vi "Get Item Data.vi"(8 "error in (no error)":errorcluster, 11 "Item Reference in":T2 format="%.0x") -> (0 "error out":errorcluster, 2 "Item Info":T1={"Name"="", "TagGUID"="", "TypeGUID"="", "Enable"=TRUE}, 3 "Item Reference out":T2 format="%.0x", 4 "found":bool)   [LabVIEW 2013, in "Hierarchy Framework.lvlib" / "Item.lvclass"]
doc: "Returns information about the item specified by <B>Item Reference in</B>, including the name of the item,and whether the item is Enable."
uses:
  Item.lvclass
  Ctls/Item Reference.ctl
  Ctls/Item Info.ctl
  Generic/Generic.lvclass
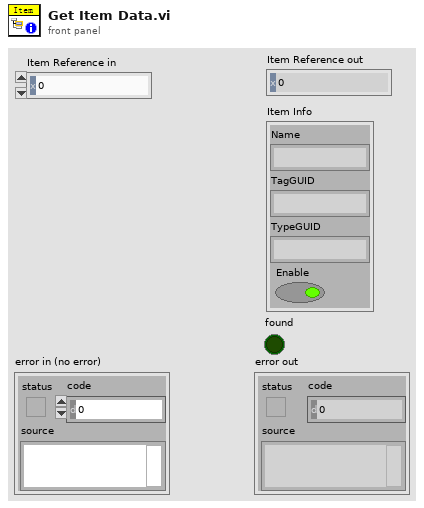
[diagram p1: front panel]
types:
  T1 = typedef "Hierarchy Framework.lvlib/Item.lvclass/Item Info.ctl" = cluster{"Name":string, "TagGUID":string, "TypeGUID":string, "Enable":bool}
  T2 = typedef "Hierarchy Framework.lvlib/Item.lvclass/Item Reference.ctl" = u64
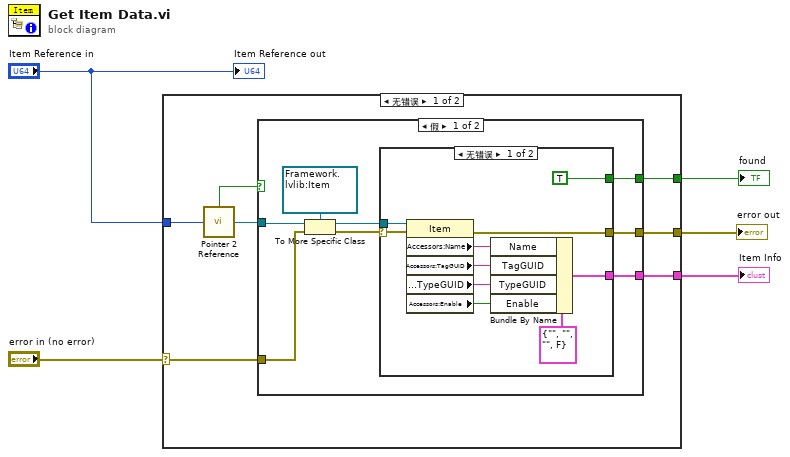
[diagram p0: block diagram]
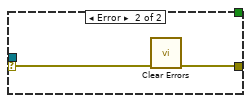
[diagram p2: hidden frame]
diagram:
  n1 = case shown="无错误" "error in (no error)" {
    selector: "error in (no error)" -> [w11 w34]
    tunnel: "Item Reference in" -> [w10 _]
    tunnel: [w12 w34] -> w4
    tunnel: [w7 _] -> w2
    tunnel: [w6 _] -> w1
    frame No Error {
      n2 = call "Pointer 2 Reference.vi"("Pointer"=w10) -> ("Not A Refnum?"=w9:bool, "Generic Reference"=w8:refnum<data-value>)
      n3 = case shown="假" w9 {
        tunnel: w11 -> [w19 w33]
        tunnel: [w16 w33] -> w12
        tunnel: w8 -> [w20 _]
        tunnel: [w15 _] -> w7
        tunnel: [w14 _] -> w6
        frame False {
          n4 = To More Specific Class(target class=refnum<data-value> refnum ("Item"), reference=w20, error in=w19) -> (specific class reference=w17:refnum<data-value>, error out=w13:errorcluster)
          n5 = case shown="无错误" w13 {
            selector: w13 -> [w21 w32]
            tunnel: w17 -> [w30 _]
            tunnel: [w29 w31] -> w16
            tunnel: [TRUE _] -> w15
            tunnel: [w23 _] -> w14
            frame No Error {
              n6 = property class="Item"(reference=w30, error in=w21) -> (error out=w29:errorcluster, "Accessors:Name"=w26:string, "Accessors:TagGUID"=w25:string, "Accessors:TypeGUID"=w22:string, "Accessors:Enable"=w24:bool)  [unwired: 1 out]
              n7 = Bundle By Name(cluster=T1 {"Name"="", "TagGUID"="", "TypeGUID"="", "Enable"=FALSE} ("Item Info"), "Name"=w26, "TagGUID"=w25, "TypeGUID"=w22, "Enable"=w24) -> (w23:T1)
            }
            frame Error {
              n8 = call <vilib>:"Clear Errors.vi"("error in (no error)"=w32) -> ("error out"=w31:errorcluster)  [unwired: 6 in]
            }
          }
        }
        frame True {
        }
      }
    }
    frame Error {
    }
  }
  "error out" <- w4
  "found" <- w2
  "Item Info" <- w1
  "Item Reference out" <- "Item Reference in"
